vi "Find Max Hysteresis.vi"(8 "error in (no error)":errorcluster, 11 "Hysteresis Points":T1[](array[typedef])) -> (0 "error out":errorcluster, 3 "Max":dbl)   [LabVIEW 2026, in "Analysis.lvlib"]
uses:
  Hysteresis Result.ctl
  Analysis.lvlib
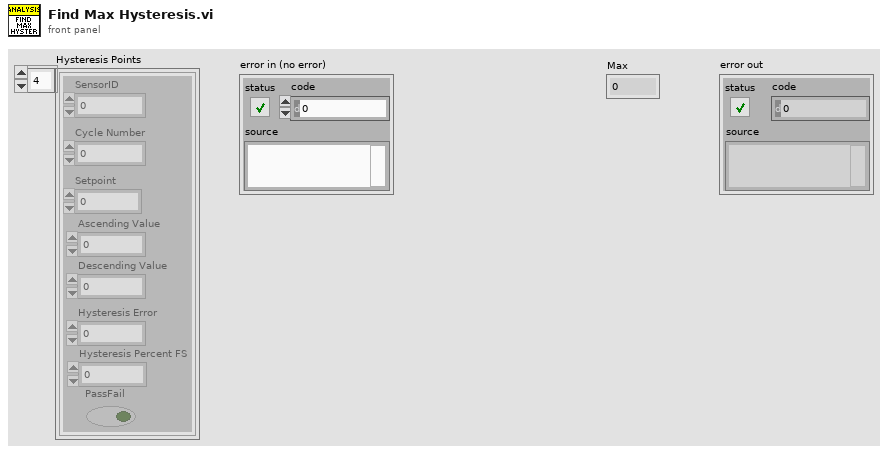
[diagram p1: front panel]
types:
  T1 = typedef "Analysis.lvlib/Hysteresis Result.ctl" = cluster{"Setpoint":dbl, "Ascending Value":dbl, "Cycle Number":i32, "SensorID":i32, "Descending Value":dbl, "Hysteresis Error":dbl, "Hysteresis Percent FS":dbl, "PassFail":bool}
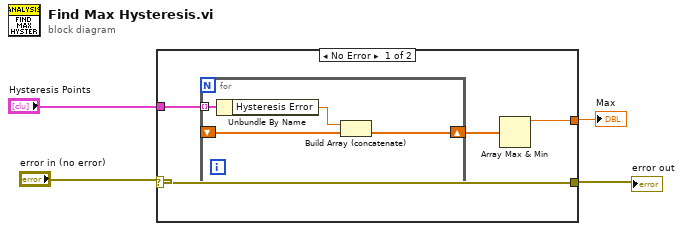
[diagram p0: block diagram]
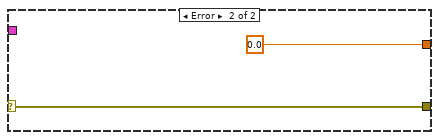
[diagram p2: hidden frame]
diagram:
  n1 = case shown="No Error" "error in (no error)" {
    selector: "error in (no error)" -> [w5 w13]
    tunnel: "Hysteresis Points" -> [w8 _]
    tunnel: [w6 0.0] -> w2
    tunnel: [w5 w13] -> w1
    frame No Error {
      n2 = for {
        tunnel: w8 -> [w12] mode=indexing
        shift-right: [w10] -> w7
        shift-left: _ -> [w9]
        n3 = Unbundle By Name(w12) -> ("Hysteresis Error"=w11:dbl)
        n4 = Build Array (concatenate)(w11, w9) -> (w10:dbl[])
      }
      n5 = Array Max & Min(array=w7) -> (max value=w6:dbl)  [unwired: 3 out]
    }
    frame Error {
    }
  }
  "error out" <- w1
  "Max" <- w2
